vi "MemoryUsage.vi"(8 "error in":errorcluster, 11 "Node Ptr":T1 format="%.0x") -> (0 "error out":errorcluster)   [LabVIEW 2026, in "SystemMonitor System Explorer.lvlib"]
uses:
  <vilib>/NI VeriStand/Custom Device API/Custom Device Item Ref.ctl
  SystemMonitor System Explorer.lvlib
  <vilib>/NI VeriStand/Custom Device API/Custom Device API.lvlib
  C:/Program Files/National Instruments/VeriStand 2026/NationalInstruments.VeriStand.Controls.dll
  Program Files/National Instruments/VeriStand 2026/NationalInstruments.VeriStand.Controls.dll
panel:
  in  "PagePropertyEditor":refnum<k24>(container)
  in  "General Header":cluster{"Section Name":string}={"Section Name"="Custom Device Section Specification"}
  in  "Description":string
  in  "Name":string
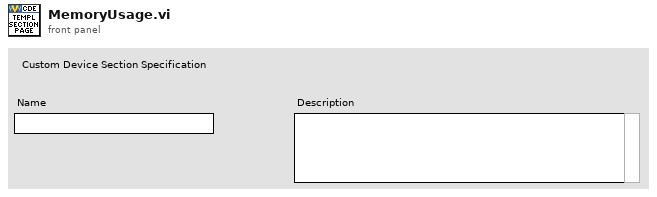
[diagram p1: front panel]
types:
  T1 = typedef "Custom Device API.lvlib/Custom Device Item Ref.ctl" = u64
  T2 = typedef "Custom Device API.lvlib/Custom Device Item Info.ctl" = cluster{"Name":string, "Is Channel":bool, "GUID":string, "Is Waveform":bool}
  T3 = typedef "Custom Device API.lvlib/Custom Device Commands.ctl" = enum16{"Default", "Item renamed", "Shutdown", "Dynamic button pressed"}
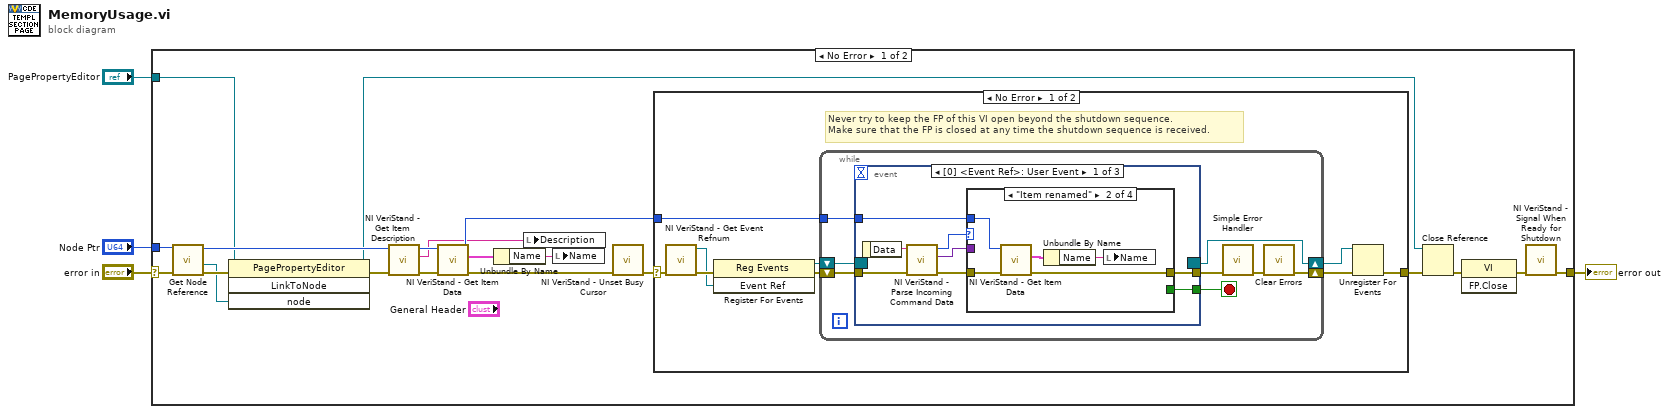
[diagram p0: block diagram]
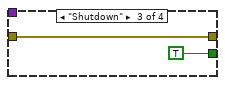
[diagram p3: hidden frame]
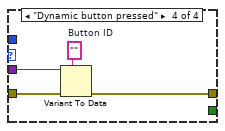
[diagram p4: hidden frame]
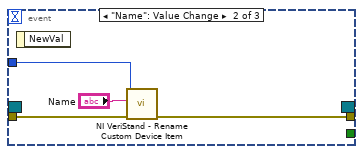
[diagram p5: hidden frame]
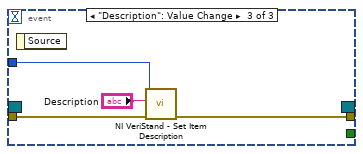
[diagram p6: hidden frame]
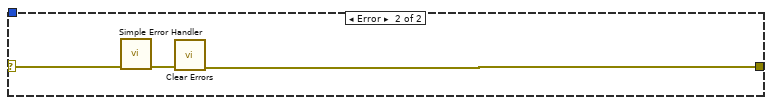
[diagram p7: hidden frame]
diagram:
  n1 = case shown="No Error" "error in" {
    selector: "error in" -> [w11 w73]
    tunnel: [w24 w73] -> w2
    tunnel: "Node Ptr" -> [w8 _]
    tunnel: "PagePropertyEditor" -> [w6 _]
    frame No Error {
      n2 = call "Get Node Reference.vi"("error in"=w11, "Node Ptr"=w8) -> ("error out"=w12:errorcluster, "Base Node"=w5:refnum<k24>, "Node Ptr"=w9:T1)  [unwired: 6 in, 1 out]
      n3 = invoke class="PagePropertyEditor" method="LinkToNode"(reference=w6, error in=w12, "node"=w5) -> (reference out=w7:refnum<k24>, error out=w10:errorcluster)  [unwired: 1 in, 2 out]
      n4 = call <vilib>:"NI VeriStand - Get Item Description.vi"("error in (no error)"=w10, "Item Ref in"=w9) -> ("error out"=w19:errorcluster, "Description"=w15:string, "Item Ref out"=w18:T1)  [unwired: 7 out]
      n5 = call <vilib>:"NI VeriStand - Get Item Data.vi"("error in (no error)"=w19, "Item Ref in"=w18) -> ("error out"=w20:errorcluster, "Item Info"=w17:T2, "Item Ref out"=w21:T1)  [unwired: 7 out]
      n6 = Unbundle By Name(w17) -> ("Name"=w16:string)
      n7 = local write "Description"(w15) -> ()
      n8 = local write "Name"(w16) -> ()
      n9 = call <vilib>:"NI VeriStand - Unset Busy Cursor.vi"("error in (no error)"=w20) -> ("error out"=w22:errorcluster)  [unwired: 10 out]
      n10 = case shown="No Error" w22 {
        selector: w22 -> [w29 w72]
        tunnel: [w31 w70] -> w14
        tunnel: w21 -> [w25 _]
        frame No Error {
          # "Never try to keep the FP of this VI open beyond the shutdown sequence.\nMake sure that the FP is closed at any time the shutdown sequence is received."
          n11 = call <vilib>:"NI VeriStand - Get Event Refnum.vi"("error in (no error)"=w29) -> ("error out"=w33:errorcluster, "Event Ref"=w27:refnum<user-event>)  [unwired: 9 out]
          n12 = register-events(error in=w33, w27) -> (reference out=w26:refnum<event-registration>, error out=w30:errorcluster)  [unwired: 1 in]
          n13 = while {
            tunnel: w25 -> [w34]
            shift-right: [w38] -> w32
            shift-left: w30 -> [w41]
            shift-right: [w37] -> w28
            shift-left: w26 -> [w36]
            stop <- w35 stop-if-true
            n14 = event shown="[0] <Event Ref>: User Event" {
              selector: w36 -> [_ _ _]
              dyn-events: [_ _ _] -> w37
              timeout: _ -> [_ _ _]
              tunnel: w41 -> [w49 w65 w69]
              tunnel: [w44 _ _] -> w35
              tunnel: [w47 w64 w68] -> w40
              tunnel: w34 -> [w43 w63 w67]
              event User Event {
                n15 = event-data() -> ("Data"=w46:string)  [unwired: 1 out]
                n16 = call <vilib>:"NI VeriStand - Parse Incoming Command Data.vi"("error in (no error)"=w49, "Incoming data"=w46) -> ("error out"=w48:errorcluster, "Outgoing data"=w42:variant, "Action"=w45:T3)  [unwired: 7 out]
                n17 = case shown="\"Item renamed\"" w45 {
                  tunnel: w48 -> [w50 w55 w57 w61]
                  tunnel: [_ _ TRUE _] -> w44
                  tunnel: [w50 w54 w57 w60] -> w47
                  tunnel: w43 -> [_ w53 _ _]
                  tunnel: w42 -> [_ _ _ w59]
                  frame "Default", Default {
                  }
                  frame "Item renamed" {
                    n18 = call <vilib>:"NI VeriStand - Get Item Data.vi"("error in (no error)"=w55, "Item Ref in"=w53) -> ("error out"=w54:errorcluster, "Item Info"=w52:T2)  [unwired: 8 out]
                    n19 = Unbundle By Name(w52) -> ("Name"=w51:string)
                    n20 = local write "Name"(w51) -> ()
                  }
                  frame "Shutdown" {
                  }
                  frame "Dynamic button pressed" {
                    w58 = ""  # Button ID
                    n21 = Variant To Data(error in=w61, type=w58, Variant=w59) -> (error out=w60:errorcluster)  [unwired: 1 out]
                  }
                }
              }
              event "Name": Value Change {
                n22 = event-data() -> ()  [unwired: 2 out]
                n23 = call <vilib>:"NI VeriStand - Rename Custom Device Item.vi"("error in (no error)"=w65, "New Name"="Name", "Item Ref in"=w63) -> ("error out"=w64:errorcluster)  [unwired: 1 in, 7 out]
              }
              event "Description": Value Change {
                n24 = event-data() -> ()  [unwired: 2 out]
                n25 = call <vilib>:"NI VeriStand - Set Item Description.vi"("error in (no error)"=w69, "Description"="Description", "Item Ref in"=w67) -> ("error out"=w68:errorcluster)  [unwired: 8 out]
              }
            }
            n26 = call <vilib>:"Simple Error Handler.vi"("error in (no error)"=w40) -> ("error out"=w39:errorcluster)  [unwired: 1 in, 7 out]
            n27 = call <vilib>:"Clear Errors.vi"("error in (no error)"=w39) -> ("error out"=w38:errorcluster)  [unwired: 1 in, 5 out]
          }
          n28 = Unregister For Events(event registration refnum=w28, error in=w32) -> (error out=w31:errorcluster)
        }
        frame Error {
          n29 = call <vilib>:"Simple Error Handler.vi"("error in (no error)"=w72) -> ("error out"=w71:errorcluster)  [unwired: 1 in, 7 out]
          n30 = call <vilib>:"Clear Errors.vi"("error in (no error)"=w71) -> ("error out"=w70:errorcluster)  [unwired: 1 in, 5 out]
        }
      }
      n31 = Close Reference(reference=w7, error in (no error)=w14) -> (error out=w13:errorcluster)
      n32 = invoke class="VI" method="FP.Close"(error in=w13) -> (error out=w23:errorcluster)  [unwired: 2 in, 2 out]
      n33 = call <vilib>:"NI VeriStand - Signal When Ready for Shutdown.vi"("error in (no error)"=w23) -> ("error out"=w24:errorcluster)  [unwired: 10 out]
    }
    frame Error {
    }
  }
  "error out" <- w2
